vi "configuration.vi"(4 "force_read?":bool, 6 "config_file":path, 7 "command":T1=enum."read_config", 8 "error in (no error)":errorcluster, 11 "config in":T2) -> (0 "error out":errorcluster, 3 "config out":T2)   [LabVIEW 2015, in "lv-builder-l3.lvlib"]
doc: "This VI is able to read/write configuration from all the associated modules defined in the master data cluster. It also acts as a functional global/data store in the event that no data has changed since the last write. It will self-initialize and well set an internal flag in the event an error is encountered when reading. If no command is provided, it will default to the read command."
uses:
  lv-builder-l3.lvlib
  public/_controls/configuration.ctl
  _controls/configuration_command.ctl
  lv-build/lv-build.lvlib
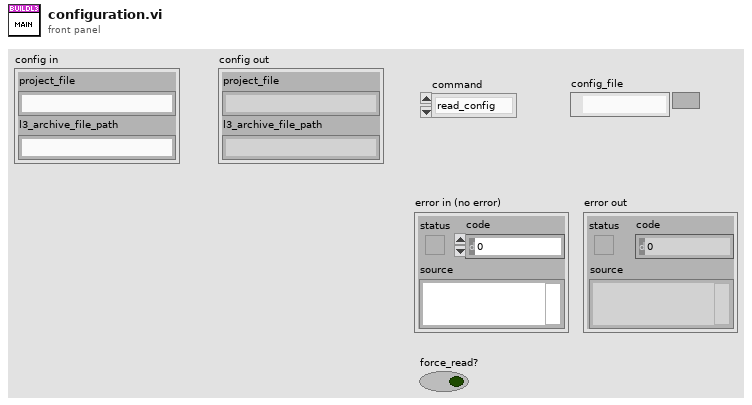
[diagram p1: front panel]
types:
  T1 = typedef "lv-builder-l3.lvlib/configuration_command.ctl" = enum16{"<config_command>", "read_config", "write_config", "<null>"}
  T2 = typedef "lv-builder-l3.lvlib/configuration.ctl" = cluster{"project_file":string, "l3_archive_file_path":string}
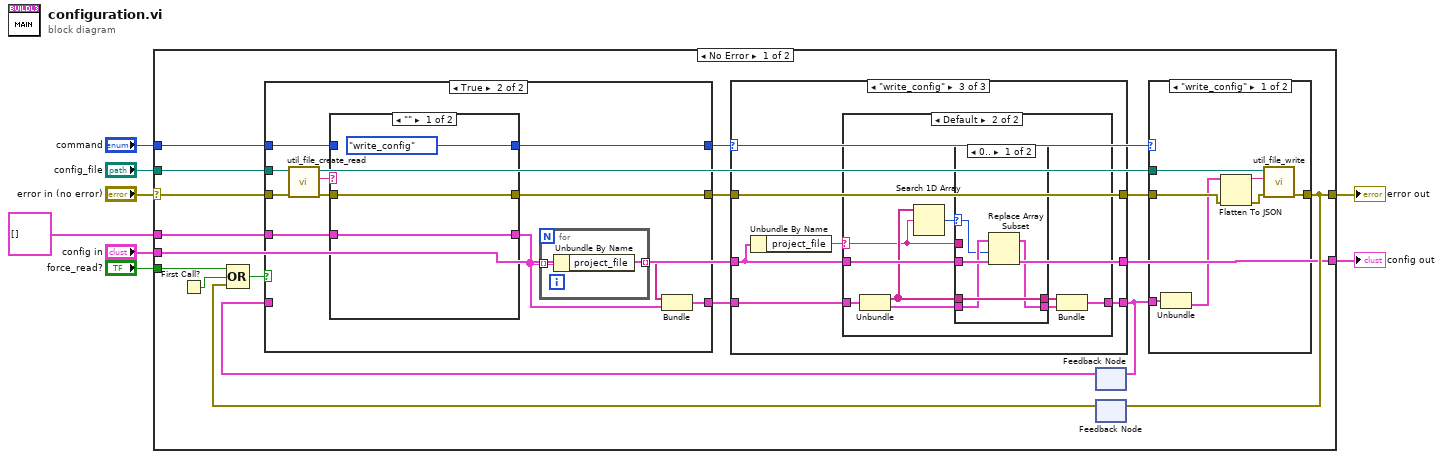
[diagram p0: block diagram]
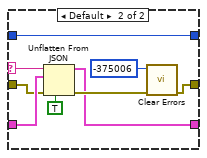
[diagram p3: hidden frame]
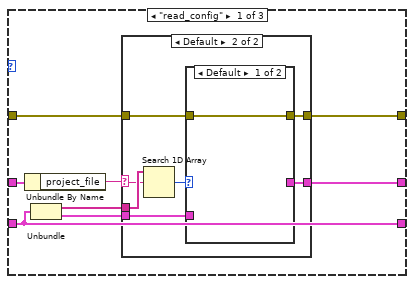
[diagram p4: hidden frame]
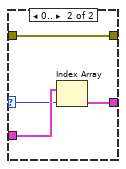
[diagram p6: hidden frame]
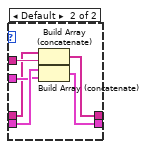
[diagram p9: hidden frame]
diagram:
  n1 = case shown="No Error" "error in (no error)" {
    selector: "error in (no error)" -> [w17 w112]
    tunnel: "command" -> [w18 _]
    tunnel: [w25 w112] -> w4
    tunnel: "config in" -> [w9 _]
    tunnel: "config_file" -> [w16 _]
    tunnel: [w10 _] -> w3
    tunnel: "force_read?" -> [w22 _]
    tunnel: T2[] [] ("default") -> [w19 _]
    frame No Error {
      n2 = First Call?() -> (First Call?: T/F=w23:bool)
      n3 = feedback #1() -> (w20:cluster{string[], "default":T2[]})  [unwired: 1 in]
      n4 = feedback #2() -> (w24:errorcluster)  [unwired: 1 in]
      n5 = Compound Arithmetic op=OR(w22, w23, w24) -> (w21:bool)
      n6 = case shown="True" w21 {
        tunnel: w20 -> [w28 _]
        tunnel: w17 -> [w27 w37]
        tunnel: w16 -> [_ w38]
        tunnel: [w27 w35] -> w14
        tunnel: w19 -> [_ w39]
        tunnel: w18 -> [w26 w34]
        tunnel: [w26 w33] -> w15
        tunnel: [w28 w29] -> w11
        frame False {
        }
        frame True {
          n7 = call "util_file_create_read.vi"("error in (no error)"=w37, "config_path"=w38) -> ("error out"=w36:errorcluster, "string"=w32:string)  [unwired: 8 in]
          n8 = case shown="\"\"" w32 {
            selector: w32 -> [_ w49]
            tunnel: w39 -> [w43 w52]
            tunnel: [w43 w51] -> w30
            tunnel: w36 -> [w44 w50]
            tunnel: [w44 w45] -> w35
            tunnel: w34 -> [_ w48]
            tunnel: [configuration_command."write_config" ("command") w48] -> w33
            frame "" {
            }
            frame Default {
              n9 = Unflatten From JSON(JSON string=w49, type and defaults=w52, default null elements? (F)=TRUE, error in (no error)=w50) -> (value=w51:T2[], error out=w53:errorcluster)  [unwired: 3 in]
              n10 = call <vilib>:"Clear Errors.vi"("error in (no error)"=w53, "specific error code to clear (0: all)"=-375006) -> ("error out"=w45:errorcluster)  [unwired: 4 in, 1 out]
            }
          }
          n11 = for {
            tunnel: w30 -> [w41] mode=indexing
            tunnel: [w40] -> w31 mode=indexing
            n12 = Unbundle By Name(w41) -> ("project_file"=w40:string)
          }
          n13 = Bundle(w31, "default"=w30) -> (w29:cluster{string[], "default":T2[]})  [unwired: 1 in]
        }
      }
      n14 = case shown="\"write_config\"" w15 {
        tunnel: w9 -> [w57 w77 w79]
        tunnel: [w61 w76 w82] -> w12
        tunnel: w11 -> [w61 w76 w80]
        tunnel: [w56 w77 w79] -> w10
        tunnel: w14 -> [w55 w75 w78]
        tunnel: [w54 w75 w78] -> w13
        frame "read_config" {
          n15 = Unbundle By Name(w57) -> ("project_file"=w58:string)
          n16 = Unbundle(w61) -> (w60:string[], "default"=w59:T2[])
          n17 = case shown="Default" w58 {
            selector: w58 -> [_ w66]
            tunnel: w60 -> [_ w69]
            tunnel: w59 -> [_ w68]
            tunnel: [_ w65] -> w56
            tunnel: w55 -> [w62 w64]
            tunnel: [w62 w63] -> w54
            frame "" {
            }
            frame Default {
              n18 = Search 1D Array(1D array=w69, element=w66) -> (index of element=w67:i32)  [unwired: 1 in]
              n19 = case shown="Default" w67 {
                selector: w67 -> [_ w73]
                tunnel: w68 -> [_ w74]
                tunnel: [_ w72] -> w65
                tunnel: w64 -> [w70 w71]
                tunnel: [w70 w71] -> w63
                frame Default {
                }
                frame 0.. {
                  n20 = Index Array(array=w74, index=w73) -> (element=w72:T2)
                }
              }
            }
          }
        }
        frame Default {
        }
        frame "write_config" {
          n21 = Unbundle By Name(w79) -> ("project_file"=w81:string)
          n22 = case shown="Default" w81 {
            selector: w81 -> [_ w84]
            tunnel: [w83 w90] -> w82
            tunnel: w79 -> [_ w88]
            tunnel: w80 -> [w83 w86]
            frame "" {
            }
            frame Default {
              n23 = Unbundle(w86) -> (w85:string[], "default"=w87:T2[])
              n24 = Search 1D Array(1D array=w85, element=w84) -> (index of element=w92:i32)  [unwired: 1 in]
              n25 = case shown="0.." w92 {
                selector: w92 -> [w93 _]
                tunnel: w87 -> [w96 w102]
                tunnel: [w95 w100] -> w91
                tunnel: w85 -> [w97 w98]
                tunnel: [w97 w99] -> w89
                tunnel: w88 -> [w94 w101]
                tunnel: w84 -> [_ w103]
                frame 0.. {
                  n26 = Replace Array Subset(array=w96, new element=w94, index=w93) -> (w95:T2[])
                }
                frame Default {
                  n27 = Build Array (concatenate)(w98, w103) -> (w99:string[])
                  n28 = Build Array (concatenate)(w102, w101) -> (w100:T2[])
                }
              }
              n29 = Bundle(w89, "default"=w91) -> (w90:cluster{string[], "default":T2[]})  [unwired: 1 in]
            }
          }
        }
      }
      n30 = feedback-in #1(w12) -> ()
      n31 = case shown="\"write_config\"" w15 {
        tunnel: w12 -> [w107 _]
        tunnel: w13 -> [w108 w111]
        tunnel: [w105 w111] -> w25
        tunnel: w16 -> [w106 _]
        frame "write_config" {
          n32 = Unbundle(w107) -> ("default"=w104:T2[])  [unwired: 1 out]
          n33 = Flatten To JSON(anything=w104, error in (no error)=w108) -> (JSON string=w110:string, 11:w109:errorcluster)  [unwired: 1 in]
          n34 = call "util_file_write.vi"("error in (no error)"=w109, "string"=w110, "config_path"=w106) -> ("error out"=w105:errorcluster)  [unwired: 8 in]
        }
        frame Default {
        }
      }
      n35 = feedback-in #2(w25) -> ()
    }
    frame Error {
      # "If an error is wired in, be sure to skip over functionality to preserve the original error"
    }
  }
  "config out" <- w3
  "error out" <- w4
